vi "Validate Metadata.vi"(8 "error in":errorcluster, 11 "measurement plugin service in":refnum<class "Measurement Plugin Service.lvclass">) -> (0 "error out":errorcluster, 3 "measurement plugin service out":refnum<class "Measurement Plugin Service.lvclass">)   [LabVIEW 2020, in "Measurement Plugin Measurement Server.lvlib"]
uses:
  Measurement Plugin Measurement Server.lvlib
  Measurement Plugin Service/Measurement Plugin Service.lvclass
  Error Strings Global Internal.vi
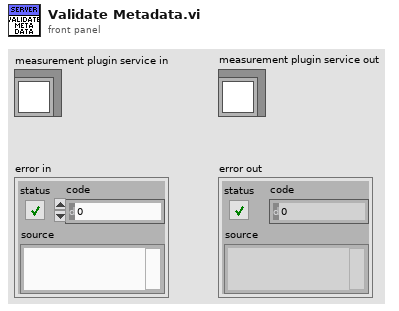
[diagram p1: front panel]
types:
  T1 = typedef "Measurement Plugin Measurement Server.lvlib/Measurement Plugin Service.lvclass/Plugin Paths.ctl" = cluster{"get measurement details VI path":path, "get type specializations VI path":path, "get UI details VI path":path, "measurement logic VI path":path, "measurement configuration ctl path":path, "measurement results ctl path":path}
  T2 = typedef "Measurement Plugin Measurement Server.lvlib/Parameter Type Specialization.ctl" = cluster{"parameter name":string, "type specialization":T3, "annotations":cluster{"key":T4, "value":string}[]}
  T3 = typedef "Measurement Plugin Measurement Server.lvlib/Type Specialization.ctl" = enum16{"none", "pin", "path", "enum", "ioresource"}
  T4 = typedef "Measurement Plugin Measurement Server.lvlib/Type Specialization Key.ctl" = enum16{"none", "pin.instrument_type", "enum.values", "ioresource.instrument_type"}
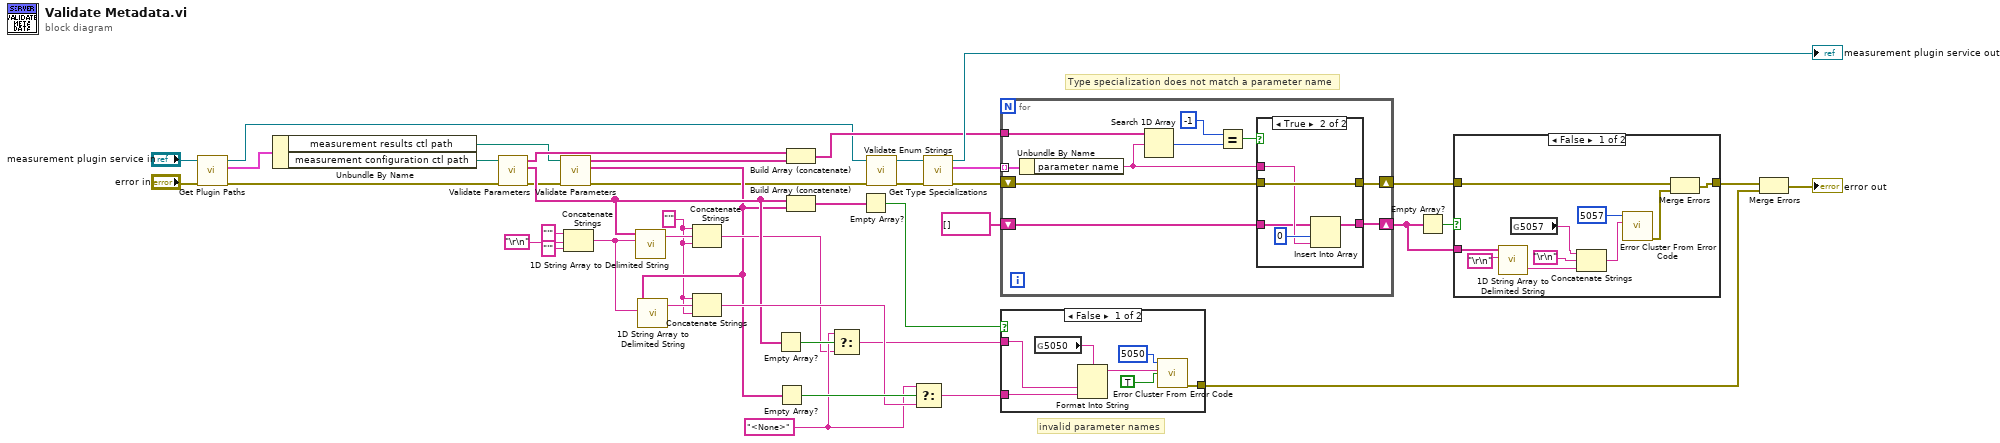
[diagram p0: block diagram]
diagram:
  w15 = "<None>" ("t")
  w1 = "'" ("string")
  # "Type specialization does not match a parameter name"
  # "invalid parameter names"
  n1 = call-dynamic "Get Plugin Paths.vi"("error in"="error in", "measurement plugin service in"="measurement plugin service in") -> ("error out"=w8:errorcluster, "plugin paths"=w37:T1, "measurement plugin service out"=w25:refnum<class "Measurement Plugin Service.lvclass">)  [unwired: 7 in]
  n2 = Unbundle By Name(w37) -> ("measurement results ctl path"=w2:path, "measurement configuration ctl path"=w3:path)
  n3 = call "Validate Parameters.vi"("error in"=w8, "path of type"=w3) -> ("error out"=w7:errorcluster, "parameters with invalid type"=w17:string[], "parameter names"=w27:string[])  [unwired: 7 in]
  n4 = call "Validate Parameters.vi"("error in"=w7, "path of type"=w2) -> ("error out"=w4:errorcluster, "parameters with invalid type"=w5:string[], "parameter names"=w6:string[])  [unwired: 7 in]
  n5 = Concatenate Strings("'" ("string"), "\r\n", "'" ("string")) -> (w9:string)
  n6 = call <vilib>:"1D String Array to Delimited String.vi"("delimiter"=w9, "string array"=w17) -> ("delimited string"=w21:string)  [unwired: 9 in]
  n7 = call <vilib>:"1D String Array to Delimited String.vi"("delimiter"=w9, "string array"=w5) -> ("delimited string"=w22:string)  [unwired: 9 in]
  n8 = Concatenate Strings(w1, w21, w1) -> (w14:string)
  n9 = Concatenate Strings(w1, w22, w1) -> (w19:string)
  n10 = Empty Array?(array=w17) -> (empty?=w16:bool)
  n11 = Empty Array?(array=w5) -> (empty?=w20:bool)
  n12 = Build Array (concatenate)(w27, w6) -> (w26:string[])
  n13 = Build Array (concatenate)(w17, w5) -> (w28:string[])
  n14 = Select(t=w15, s=w16, f=w14) -> (s? t:f=w13:string)
  n15 = Empty Array?(array=w28) -> (empty?=w32:bool)
  n16 = call "Validate Enum Strings.vi"("error in"=w4, "measurement plugin service in"=w25) -> ("error out"=w23:errorcluster, "measurement plugin service out"=w24:refnum<class "Measurement Plugin Service.lvclass">)  [unwired: 8 in]
  n17 = Select(t=w15, s=w20, f=w19) -> (s? t:f=w18:string)
  n18 = call-dynamic "Get Type Specializations.vi"("error in"=w23, "measurement plugin service in"=w24) -> ("error out"=w41:errorcluster, "type specializations"=w40:T2[], "measurement plugin service out"=→"measurement plugin service out":refnum<class "Measurement Plugin Service.lvclass">)  [unwired: 7 in]
  n19 = for {
    tunnel: w40 -> [w52] mode=indexing
    shift-right: [w48] -> w33
    shift-left: w41 -> [w49]
    tunnel: w26 -> [w51]
    shift-right: [w45] -> w36
    shift-left: string[] [] -> [w47]
    n20 = Unbundle By Name(w52) -> ("parameter name"=w46:string)
    n21 = Search 1D Array(1D array=w51, element=w46) -> (index of element=w43:i32)  [unwired: 1 in]
    n22 = Equal?(x=-1 ("y"), y=w43) -> (x = y?=w50:bool)
    n23 = case shown="True" w50 {
      tunnel: w49 -> [w54 w59]
      tunnel: [w54 w59] -> w48
      tunnel: w47 -> [w53 w56]
      tunnel: w46 -> [_ w57]
      tunnel: [w53 w55] -> w45
      frame False {
      }
      frame True {
        n24 = Insert Into Array(array=w56, index=0, new element=w57) -> (w55:string[])
      }
    }
  }
  n25 = case shown="False" w32 {
    tunnel: [w66 _] -> w29
    tunnel: w13 -> [w63 _]
    tunnel: w18 -> [w60 _]
    frame False {
      n26 = global read "Error Strings Global Internal.vi" "5050"() -> (w61:string)
      n27 = Format Into String(format string=w61, w63, w60) -> (resulting string=w62:string)  [unwired: 2 in, 1 out]
      n28 = call <vilib>:"Error Cluster From Error Code.vi"("show call chain? (False)"=TRUE, "error message (\"\")"=w62, "error code (0)"=5050) -> ("error out"=w66:errorcluster)  [unwired: 6 in]
    }
    frame True {
    }
  }
  n29 = Empty Array?(array=w36) -> (empty?=w35:bool)
  n30 = case shown="False" w35 {
    tunnel: w36 -> [w73 _]
    tunnel: w33 -> [w68 w77]
    tunnel: [w69 w77] -> w30
    frame False {
      n31 = call <vilib>:"1D String Array to Delimited String.vi"("delimiter"="\r\n", "string array"=w73) -> ("delimited string"=w74:string)  [unwired: 9 in]
      n32 = global read "Error Strings Global Internal.vi" "5057"() -> (w72:string)
      n33 = Concatenate Strings(w72, "\r\n", w74) -> (w70:string)
      n34 = call <vilib>:"Error Cluster From Error Code.vi"("error message (\"\")"=w70, "error code (0)"=5057) -> ("error out"=w67:errorcluster)  [unwired: 7 in]
      n35 = Merge Errors(w68, w67) -> (w69:errorcluster)
    }
    frame True {
    }
  }
  n36 = Merge Errors(w30, w29) -> (→"error out":errorcluster)
